vi "Get PortID.vi"() -> (2 "PortID":u16)   [LabVIEW 2020, in "FlexLogger_gRPC.lvlib" / "FlexLogger_gRPC.lvclass"]
uses:
  FlexLogger_gRPC.lvclass
  <vilib>/Utility/sysdir.llb/System Directory Type.ctl
  FlexLogger_gRPC.lvclass/FlexLogger_gRPC.ctl
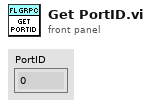
[diagram p1: front panel]
types:
  T1 = typedef "System Directory Type.ctl" = i32
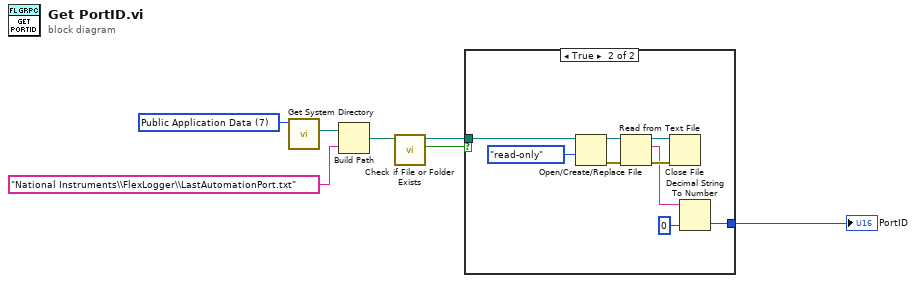
[diagram p0: block diagram]
diagram:
  w7 = T1 7 items=["User Home"=0, "User Desktop"=1, "User Documents"=2, "User Application Data"=3, "User Preferences"=4, "User Temporary"=5, "Public Documents"=6, "Public Application Data"=7, "Public Preferences"=8, "Public Cache"=13, "System Core Libraries"=9, "System Installed Libraries"=10, "Application Files"=11, "Boot Volume Root"=12] ("system directory type")
  n1 = call <vilib>:"Get System Directory.vi"("system directory type"=w7) -> ("system directory"=w6:path)  [unwired: 10 in]
  n2 = Build Path(base path=w6, name or relative path="National Instruments\\FlexLogger\\LastAutomationPort.txt") -> (appended path=w2:path)
  n3 = call <vilib>:"Check if File or Folder Exists.vi"("path"=w2) -> ("file or folder exists?"=w3:bool, "dup path"=w1:path)  [unwired: 8 in, 1 out]
  n4 = case shown="True" w3 {
    tunnel: [_ w11] -> w4
    tunnel: w1 -> [_ w9]
    frame False {
    }
    frame True {
      n5 = Open/Create/Replace File(file path (use dialog)=w9, access (0:read/write)=enum16{"read/write", "read-only", "write-only"}."read-only") -> (refnum out=w15:refnum<file>, error out=w16:errorcluster)  [unwired: 4 in, 1 out]
      n6 = Read from Text File(file (use dialog)=w15, error in=w16) -> (refnum out=w13:refnum<file>, text=w12:string, error out=w14:errorcluster)  [unwired: 2 in, 1 out]
      n7 = Close File(refnum=w13, error in=w14) -> ()  [unwired: 2 out]
      n8 = Decimal String To Number(string=w12, default (0L)=u16 0 ("default (0 I32)")) -> (number=w11:u16)  [unwired: 1 in, 1 out]
    }
  }
  "PortID" <- w4
